vi "Enum to Gain.vi"(1 "Gain":T1) -> (0 "Gain (x)":dbl)   [LabVIEW 2019, in "KH7008.lvlib"]
uses:
  KH7008.lvlib
  typedefs/gain--enum.ctl
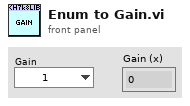
[diagram p1: front panel]
types:
  T1 = typedef "KH7008.lvlib/gain--enum.ctl" = enum16{"1", "10", "100", "1000"}
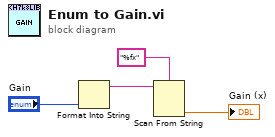
[diagram p0: block diagram]
diagram:
  n1 = Format Into String("Gain") -> (resulting string=w1:string)  [unwired: 3 in, 1 out]
  n2 = Scan From String(format string="%fx", input string=w1) -> (output 1=→"Gain (x)":dbl)  [unwired: 3 in, 3 out]
